vi "Configure All Results Enabled.vi"(8 "error in (no error)":errorcluster, 9 "Enable All Results":bool[](array[boolean]), 10 "Instance (1)":T1=1, 11 "VISA resource name":refnum<visa-resource-name>) -> (0 "error out":errorcluster, 3 "VISA resource name out":refnum<visa-resource-name>)   [LabVIEW 2020, in "Rohde&Schwarz CMWXP NR FR1 Measurement.lvlib"]
doc: "Enables or disables the evaluation of results in the multi-evaluation measurement. This command combines most other CONFigure:NRSub:MEAS<i>:MEValuation:RESult... commands.\n\nAttribute:\nRSCMWXPNRFR1M_ATTR_ALL_RESULTS_ENABLED\n\nRemote-control command:\nCONFigure:NRSub:MEAS<i>:MEValuation:RESult[:ALL]"
uses:
  <instrlib>/Rohde&Schwarz CMWXP NR FR1 Measurement/Rohde&Schwarz CMWXP NR FR1 Measurement.lvlib
  <instrlib>/Rohde&Schwarz CMWXP NR FR1 Measurement/Private/_Instance.ctl
  <instrlib>/Rohde&Schwarz CMWXP NR FR1 Measurement/Private/rsidr_core.llb/rsidr_core.lvlib
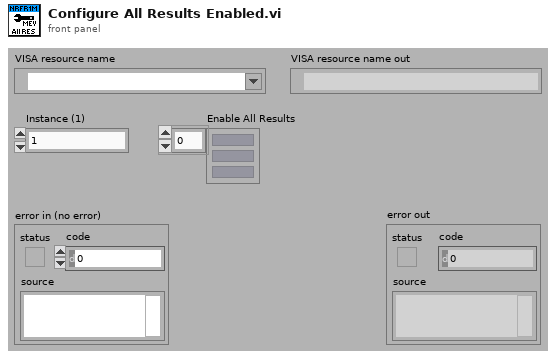
[diagram p1: front panel]
types:
  T1 = typedef "Rohde&Schwarz CMWXP NR FR1 Measurement.lvlib/_Instance.ctl" = i32
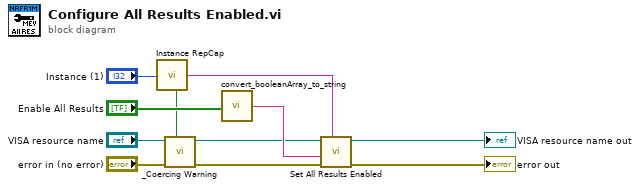
[diagram p0: block diagram]
diagram:
  n1 = call <instrlib>:"Instance RepCap.vi"("Instance In"="Instance (1)") -> ("In Range?"=w1:bool, "RepCap Identifier Out"=w8:string)  [unwired: 1 in]
  n2 = call <instrlib>:"_Coercing Warning.vi"("In Range?"=w1, "error in (no error)"="error in (no error)", "VISA resource name"="VISA resource name") -> ("error out"=w3:errorcluster, "VISA resource name out"=w2:refnum<visa-resource-name>)  [unwired: 7 in]
  n3 = call <instrlib>:"convert_booleanArray_to_string.vi"("Boolean array in"="Enable All Results") -> ("string out"=w6:string)  [unwired: 4 in]
  n4 = call "Set All Results Enabled"("Repeated Capabilities"=w8, "error in (no error)"=w3, "All Results Enabled ()"=w6, "instrument handle"=w2) -> ("error out"=→"error out":errorcluster, "instrument handle out"=→"VISA resource name out":refnum<visa-resource-name>)  [unwired: 6 in]
